vi "Read Configuration Data.vi"(8 "error in (no error)":errorcluster) -> (0 "error out":errorcluster, 3 "MHL Configuration":T1)   [LabVIEW 2015]
uses:
  controls/MHL Configuration.ctl
  Boiler System Globals.vi
  <vilib>/Utility/config.llb/NI_LVConfig.lvlib
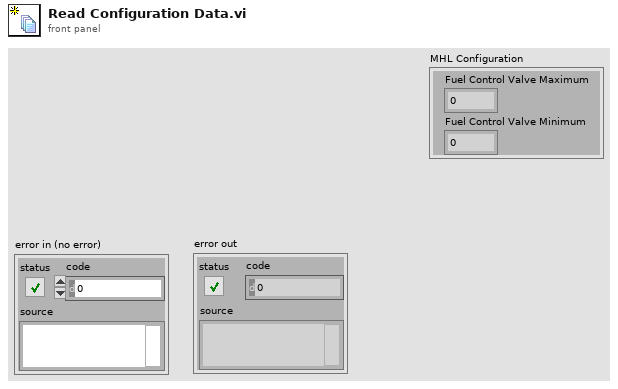
[diagram p1: front panel]
types:
  T1 = typedef "MHL Configuration.ctl" = cluster{"Fuel Control Valve Maximum":dbl, "Fuel Control Valve Minimum":dbl}
  T2 = typedef "NI_LVConfig.lvlib/Config Data RefNum.ctl" = refnum<k1>
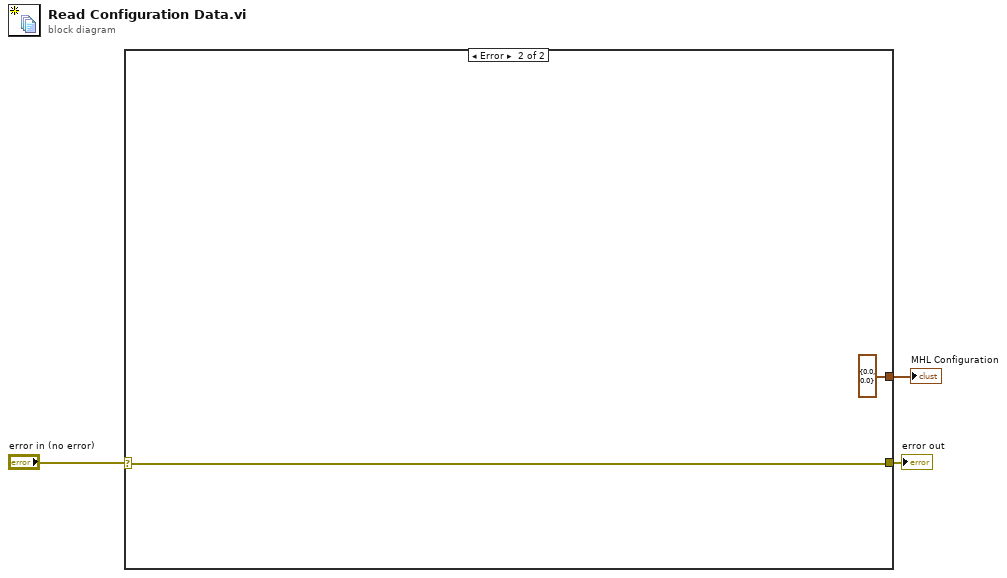
[diagram p0: block diagram]
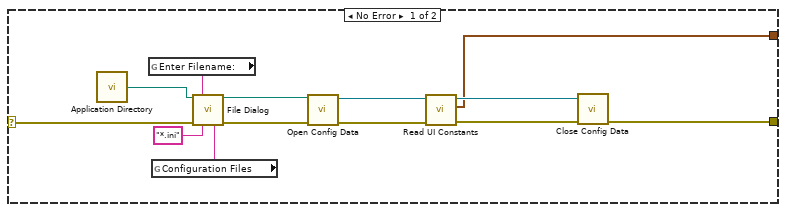
[diagram p2: hidden frame]
diagram:
  n1 = case shown="Error" "error in (no error)" {
    selector: "error in (no error)" -> [w16 w17]
    tunnel: [w10 w17] -> w2
    tunnel: [w4 T1 {"Fuel Control Valve Maximum"=0.0, "Fuel Control Valve Minimum"=0.0} ("MHL Configuration")] -> w1
    frame No Error {
      n2 = call <vilib>:"Application Directory.vi"() -> ("Application Directory"=w12:path)
      n3 = global read "Boiler System Globals.vi" "Enter Filename:"() -> (w13:string)
      n4 = global read "Boiler System Globals.vi" "Configuration Files"() -> (w14:string)
      n5 = call "File Dialog"("start path"=w12, "prompt"=w13, "error in"=w16, "pattern (all files)"="*.ini", "pattern label"=w14) -> ("selected path"=w7:path, "error out"=w8:errorcluster)  [unwired: 7 in, 2 out]
      n6 = call <vilib>:"Open Config Data.vi"("error in (no error)"=w8, "configuration file path"=w7) -> ("error out"=w9:errorcluster, "refnum"=w6:T2)  [unwired: 7 in, 1 out]
      n7 = call "Read UI Constants.vi"("error in (no error)"=w9, "CFG File Refnum in"=w6) -> ("error out"=w11:errorcluster, "MHL Configuration"=w4:T1, "CFG File Refnum out"=w5:T2)  [unwired: 7 in]
      n8 = call <vilib>:"Close Config Data.vi"("error in (no error)"=w11, "refnum"=w5) -> ("error out"=w10:errorcluster)  [unwired: 8 in, 1 out]
    }
    frame Error {
    }
  }
  "error out" <- w2
  "MHL Configuration" <- w1
